vi "red laser.vi"(8 "error in (no error)":errorcluster) -> (0 "error out":errorcluster, 3 "IR":dbl[](array[numeric]))   [LabVIEW 2018]
uses:
  <vilib>/Utility/error.llb/Error Cluster From Error Code.vi
  <vilib>/myRIO/Common/Instrument Driver Framework/myRIO v1.0/AI/vis/myRIO v1.0 Read AI.vi
  <vilib>/myRIO/Instrument Drivers/Onboard IO/AI/AI.lvlib
panel:
  out "chin":dbl
  out "ho":dbl
  out "left":dbl
  out "right":dbl
  out "B/AI0 (Pin 3)":dbl
  out "B/AI1 (Pin 5)":dbl
  out "B/AI2 (Pin 7)":dbl
  out "B/AI3 (Pin 9)":dbl
  out "C/AI0 (AI0)":dbl
  out "C/AI1 (AI1)":dbl
  in  "stop":bool
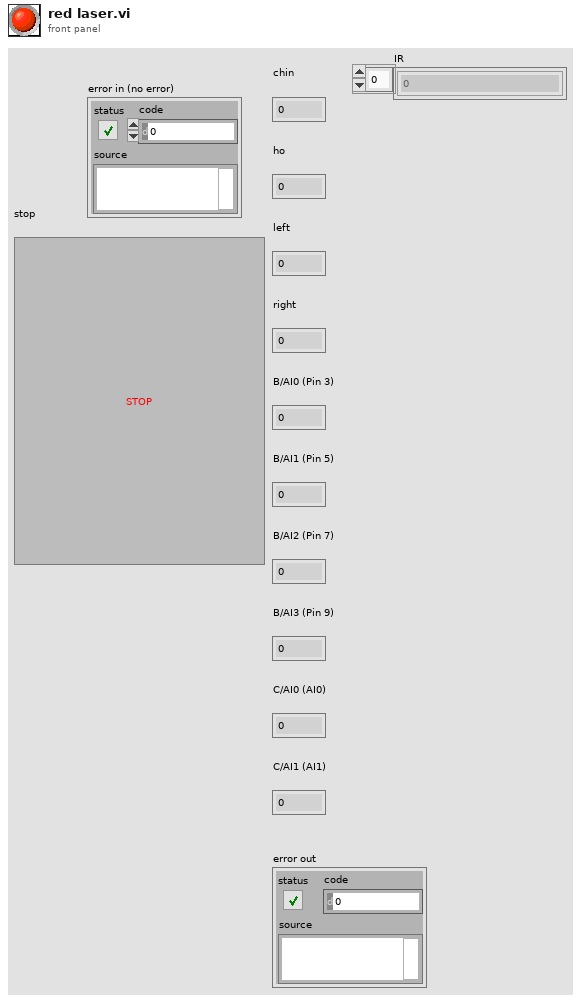
[diagram p1: front panel]
types:
  T1 = typedef "AI.lvlib/AI Reference.ctl" = cluster{"myRIO Reference":T2, "AI Channels List":T6, "AI Scaling Constants List":T8}
  T2 = typedef "myRIO Generic Hardware Reference.ctl" = cluster{"myRIO Model":T3, "myRIO Hardware Reference":T4}
  T3 = typedef "Hardware Version Enum.ctl" = enum16{"Unknown", "myRIO-1900", "myRIO-1950", "roboRIO", "NI ELVIS RIO CM", "ELVIS III"}
  T4 = typedef "myRIO v1.0 Reference.ctl" = cluster{"Generic FPGA Reference":T5, "Allow multiple opens":bool}
  T5 = typedef "Generic FPGA Reference.ctl" = refnum<k20>
  T6 = typedef "AI Channels List.ctl" = T7[]
  T7 = typedef "AI Channels Enum.ctl" = enum16{"Not Connected", "AudioIn/Left", "AudioIn/Right", "C/AI0", "C/AI1", "A/AI0", "A/AI1", "A/AI2", "A/AI3", "A/AI4", "A/AI5", "A/AI6", "A/AI7", "B/AI0", "B/AI1", "B/AI2", "B/AI3", "B/AI4", "B/AI5", "B/AI6", "B/AI7", "AI/AI0", "AI/AI1", "AI/AI2", "AI/AI3", "A/AI0 (DIFF)", "A/AI1 (DIFF)", "A/AI2 (DIFF)", "A/AI3 (DIFF)", "B/AI0 (DIFF)", "B/AI1 (DIFF)", "B/AI2 (DIFF)", "B/AI3 (DIFF)"}
  T8 = typedef "Analog Scaling Constants List.ctl" = T9[]
  T9 = typedef "Analog Scaling Constants.ctl" = cluster{"LSB Weight (Volts)":dbl, "Offset (Volts)":dbl, "Signed?":bool}
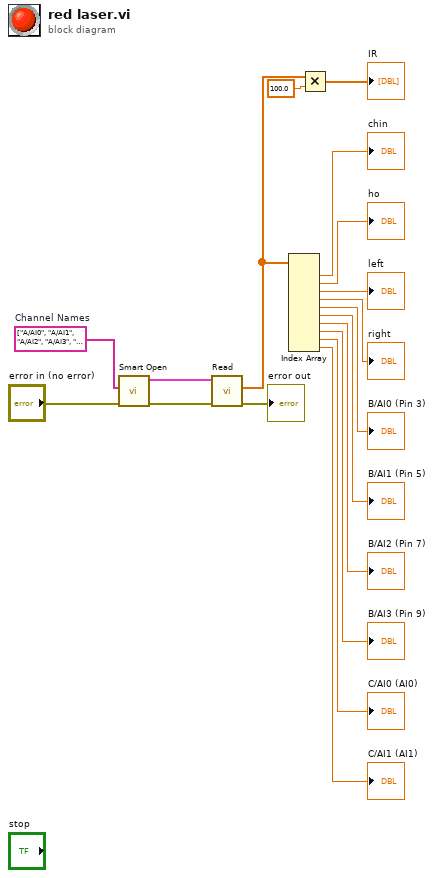
[diagram p0: block diagram]
diagram:
  w18 = tag[] ["A/AI0", "A/AI1", "A/AI2", "A/AI3", "B/AI0", "B/AI1", "B/AI2", "B/AI3", "C/AI0", "C/AI1"]  # Channel Names
  n1 = call <vilib>:"Smart Open.vi"("error in (no error)"="error in (no error)", "Channel Names"=w18) -> ("error out"=w7:errorcluster, "AI Ref Out"=w8:T1)  [unwired: 8 in]
  n2 = call <vilib>:"Read.vi"("error in (no error)"=w7, "AI Ref In"=w8) -> ("error out"=→"error out":errorcluster, "Values"=w2:dbl[])  [unwired: 7 in, 1 out]
  n3 = Index Array(array=w2) -> (element #1=→"chin":dbl, element #2=→"ho":dbl, element #3=→"left":dbl, element #4=→"right":dbl, element #5=→"B/AI0 (Pin 3)":dbl, element #6=→"B/AI1 (Pin 5)":dbl, element #7=→"B/AI2 (Pin 7)":dbl, element #8=→"B/AI3 (Pin 9)":dbl, element #9=→"C/AI0 (AI0)":dbl, element #10=→"C/AI1 (AI1)":dbl)  [unwired: 10 in]
  n4 = Multiply(x=w2, y=100.0) -> (x*y=→"IR":dbl[])
